vi "Open Bus Monitor.vi"(8 "error in (no error)":errorcluster, 11 "IMediator in":refnum<class "IMediator.lvclass">) -> (0 "error out":errorcluster, 3 "IMediator out":refnum<class "IMediator.lvclass">)   [LabVIEW 2015, in "IMediator.lvlib" / "IMediator.lvclass"]
uses:
  IMediator.lvclass
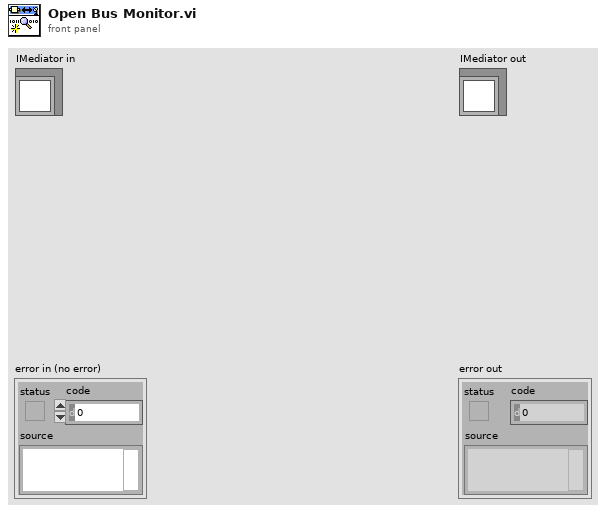
[diagram p1: front panel]
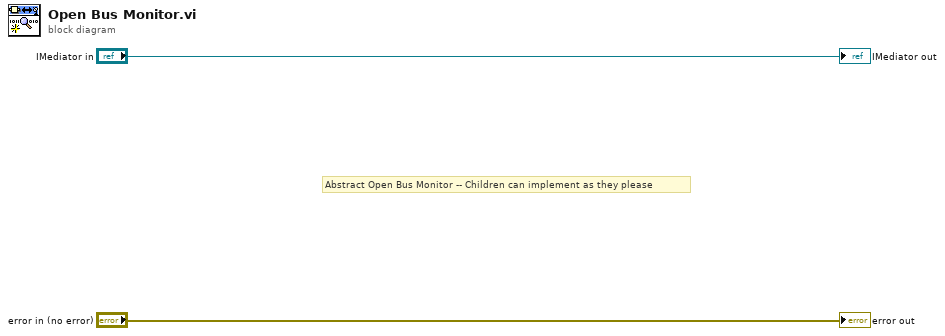
[diagram p0: block diagram]
diagram:
  # "Abstract Open Bus Monitor -- Children can implement as they please"
  "error out" <- "error in (no error)"
  "IMediator out" <- "IMediator in"
